vi "ziAutoRange.vi"(8 "Error in":errorcluster, 10 "Path":string, 11 "Handle in":T1 {"Handle" format="0x%08x"; "Conn" format="0x%08x"}) -> (0 "Error out":errorcluster, 1 "Success":bool, 3 "Handle out":T1 {"Handle" format="0x%08x"; "Conn" format="0x%08x"})   [LabVIEW 2009, in "Zurich Instruments LabOne.lvlib"]
doc: "Automatically set the input range of signalinputs/{0,1} to half full level.\n<B>Path</B> can either be sigins/0 or sigins/1"
uses:
  <instrlib>/Zurich Instruments LabOne/Zurich Instruments LabOne.lvlib
  <instrlib>/Zurich Instruments LabOne/Public/ziTypeHandle.ctl
  <instrlib>/Zurich Instruments LabOne/Public/Configure/ziGetValueString.vi
  <vilib>/regexp/Match Regular Expression.xnode
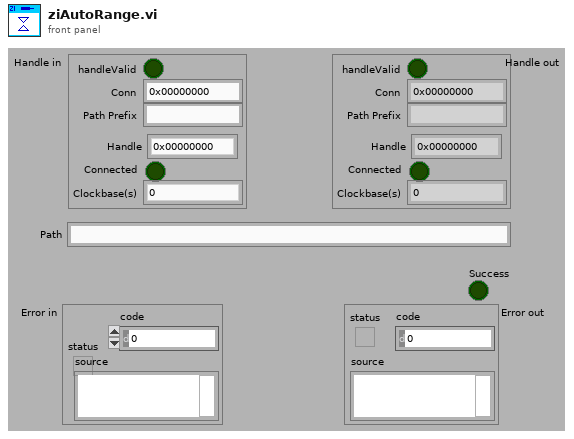
[diagram p1: front panel]
types:
  T1 = typedef "Zurich Instruments LabOne.lvlib/ziTypeHandle.ctl" = cluster{"handleValid":bool, "Conn":u64, "Path Prefix":string, "Handle":u64, "Connected":bool, "Clockbase(s)":dbl}
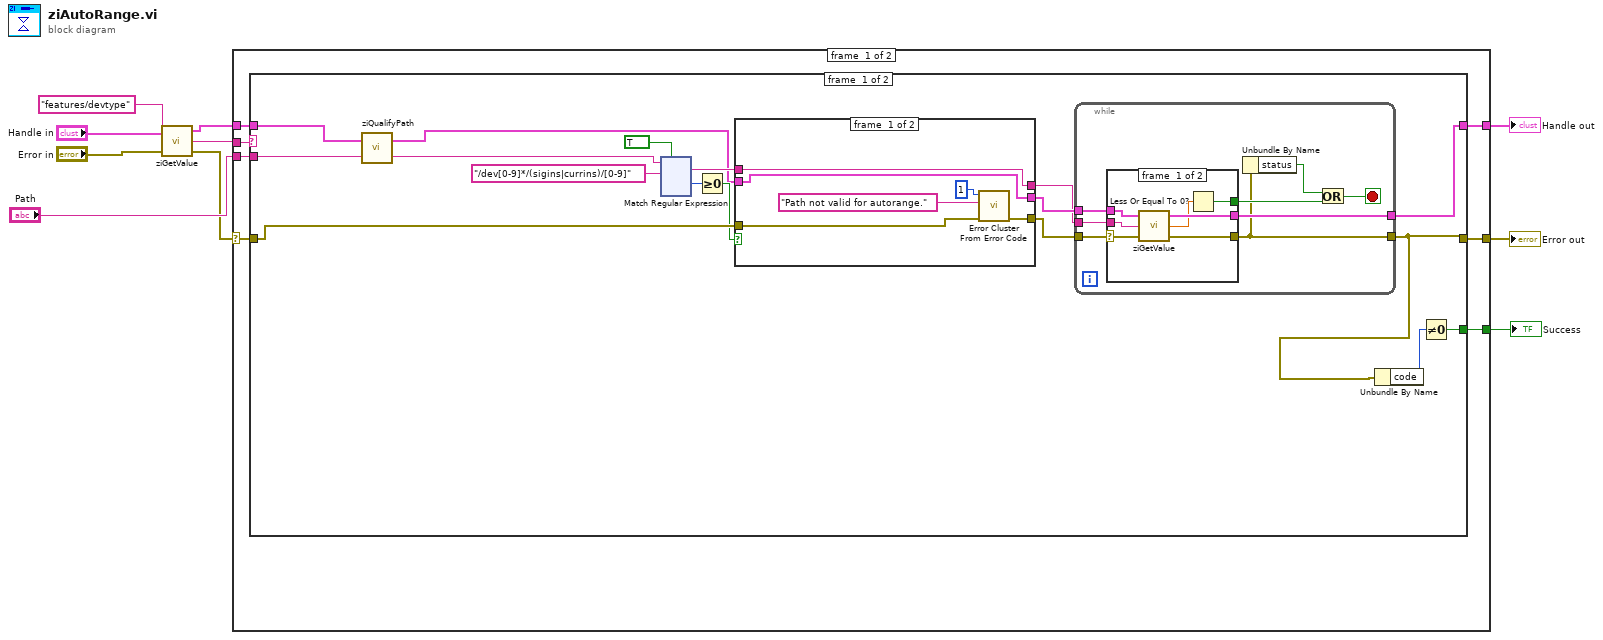
[diagram p0: block diagram]
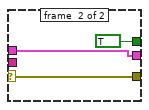
[diagram p2: hidden frame]
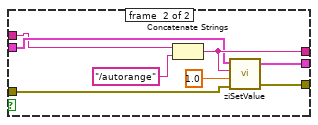
[diagram p3: hidden frame]
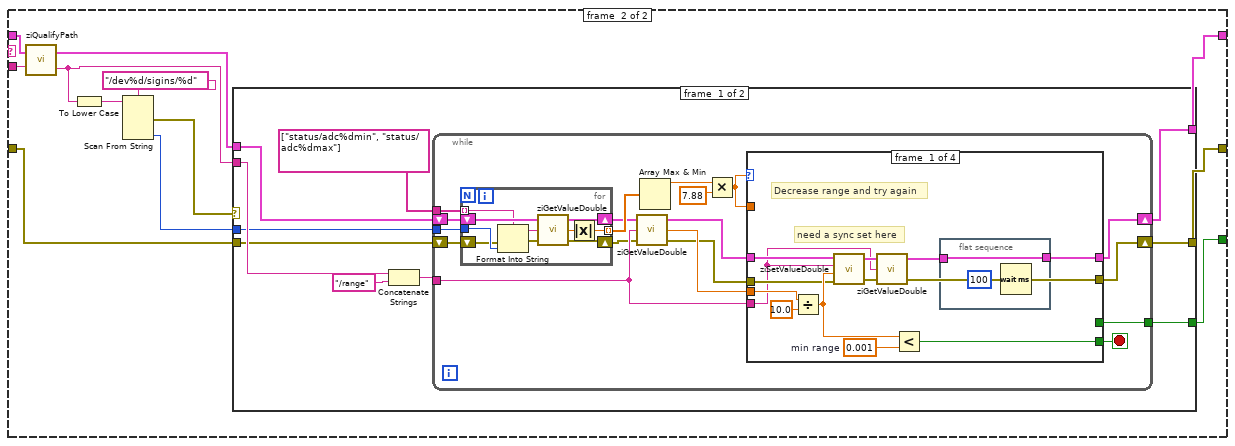
[diagram p4: hidden frame]
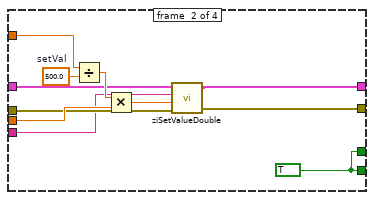
[diagram p5: hidden frame]
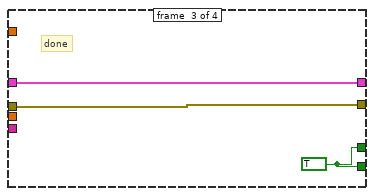
[diagram p6: hidden frame]
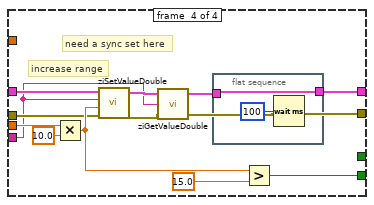
[diagram p7: hidden frame]
diagram:
  n1 = call-poly <instrlib>:"ziGetValue.vi"("error in"="Error in", "Path"="features/devtype", "Handle In"="Handle in") -> ("error out"=w2:errorcluster, "Value"=w1:string, "Handle Out"=w3:T1)
  n2 = case shown="No Error" w2 {
    selector: w2 -> [w15 w270]
    tunnel: [w17 w270] -> w10
    tunnel: [w16 w271] -> w9
    tunnel: w3 -> [w13 w271]
    tunnel: "Path" -> [w14 _]
    tunnel: [w12 _] -> w7
    tunnel: w1 -> [w11 _]
    frame #0 {
      n3 = case shown="Default" w11 {
        tunnel: [w18 w185] -> w17
        tunnel: [w32 w184] -> w16
        tunnel: w15 -> [w34 w183]
        tunnel: w14 -> [w23 w182]
        tunnel: w13 -> [w24 w181]
        tunnel: [w20 w177] -> w12
        frame #0 {
          n4 = call <instrlib>:"ziQualifyPath.vi"("Path In"=w23, "Handle In"=w24) -> ("Path Out"=w19:string, "Handle Out"=w22:T1)
          n5 = xnode "Match Regular Expression"("input string"=w19, "regular expression"="/dev[0-9]*/(sigins|currins)/[0-9]", "ignore case? (F)"=TRUE) -> ("whole match"=w29:string, "offset past match"=w27:i32)  [unwired: 3 in, 3 out]
          n6 = Greater Or Equal To 0?(x=w27) -> (x >= 0?=w28:bool)
          n7 = case shown="True" w28 {
            tunnel: w34 -> [w163 w173]
            tunnel: w22 -> [w165 w167]
            tunnel: [w165 w170] -> w33
            tunnel: [w164 w169] -> w31
            tunnel: [w162 w168] -> w30
            tunnel: w29 -> [w164 w166]
            frame #0 {
              n8 = call <vilib>:"Error Cluster From Error Code.vi"("error in (no error)"=w163, "error message (\"\")"="Path not valid for autorange." ("error message (\"\")"), "error code (0)"=1) -> ("error out"=w162:errorcluster)  [unwired: 6 in]
            }
            frame #1 {
              n9 = Concatenate Strings(w166, "/autorange") -> (w169:string)
              n10 = call-poly <instrlib>:"ziSetValue.vi"("Error In"=w173, "Value"=1.0, "Path"=w169, "Handle In"=w167) -> ("Error Out"=w168:errorcluster, "Handle Out"=w170:T1)  [unwired: 1 in]
            }
          }
          n11 = while {
            tunnel: w30 -> [w39]
            tunnel: w33 -> [w42]
            tunnel: [w41] -> w32
            tunnel: w31 -> [w40]
            tunnel: [w37] -> w18
            stop <- w35 stop-if-true
            n12 = case shown="No Error" w39 {
              selector: w39 -> [w43 w51]
              tunnel: w42 -> [w49 w52]
              tunnel: [w48 w52] -> w41
              tunnel: w40 -> [w47 _]
              tunnel: [w46 TRUE] -> w38
              tunnel: [w44 w51] -> w37
              frame #0 {
                n13 = call-poly <instrlib>:"ziGetValue.vi"("error in"=w43, "Path"=w47, "Handle in"=w49) -> ("error out"=w44:errorcluster, "Value"=w45:dbl, "Handle out"=w48:T1)
                n14 = Less Or Equal To 0?(x=w45) -> (x <= 0?=w46:bool)
              }
              frame #1 {
              }
            }
            n15 = Unbundle By Name(w37) -> ("status"=w36:bool)
            n16 = Or(x=w36, y=w38) -> (x .or. y?=w35:bool)
          }
          n17 = Unbundle By Name(w18) -> ("code"=w21:i32)
          n18 = Not Equal To 0?(x=w21) -> (x != 0?=w20:bool)
        }
        frame #1 {
          n19 = call <instrlib>:"ziQualifyPath.vi"("Path In"=w182, "Handle In"=w181) -> ("Path Out"=w176:string, "Handle Out"=w180:T1)
          n20 = To Lower Case(string=w176) -> (all lower case string=w175:string)
          n21 = Scan From String(format string="/dev%d/sigins/%d" ("regular expression"), input string=w175) -> (error out=w179:errorcluster, output 2=w174:i32)  [unwired: 5 in, 2 out]
          n22 = case shown="No Error" w179 {
            tunnel: [w192 w269] -> w185
            tunnel: [w193 w268] -> w184
            tunnel: w180 -> [w194 w268]
            tunnel: w183 -> [w186 w269]
            tunnel: w176 -> [w189 _]
            tunnel: w174 -> [w187 _]
            tunnel: [w188 _] -> w177
            frame #0 {
              n23 = Concatenate Strings(w189, "/range") -> (w191:string)
              n24 = while {
                shift-right: [w210] -> w193
                shift-left: w194 -> [w206]
                shift-right: [w209] -> w192
                shift-left: w186 -> [w198]
                tunnel: w191 -> [w201]
                tunnel: string[] ["status/adc%dmin", "status/adc%dmax"] -> [w205]
                tunnel: w187 -> [w197]
                tunnel: [w196] -> w188
                stop <- w208 stop-if-true
                n25 = for {
                  tunnel: w205 -> [w218] mode=indexing
                  tunnel: [w223] -> w213 mode=indexing
                  shift-right: [w222] -> w204
                  shift-left: w206 -> [w221]
                  tunnel: w197 -> [w217]
                  shift-right: [w219] -> w199
                  shift-left: w198 -> [w215]
                  n26 = Format Into String(format string=w218, error in=w215, w217) -> (resulting string=w216:string, error out=w214:errorcluster)  [unwired: 1 in]
                  n27 = call <instrlib>:"ziGetValueDouble.vi"("error in"=w214, "Path"=w216, "Handle in"=w221) -> ("error out"=w219:errorcluster, "Value"=w220:dbl, "Handle out"=w222:T1)
                  n28 = Absolute Value(x=w220) -> (abs(x)=w223:dbl)
                }
                n29 = call <instrlib>:"ziGetValueDouble.vi"("error in"=w199, "Path"=w201, "Handle in"=w204) -> ("error out"=w200:errorcluster, "Value"=w202:dbl, "Handle out"=w203:T1)
                n30 = Array Max & Min(array=w213) -> (max value=w211:dbl)  [unwired: 3 out]
                n31 = Multiply(x=w211, y=7.88 ("valueD")) -> (x*y=w207:dbl)
                n32 = case shown="1000..10000" w207 {
                  tunnel: w203 -> [w233 w243 w251 w261]
                  tunnel: w200 -> [w231 w241 w252 w259]
                  tunnel: [w226 w245 w251 w255] -> w210
                  tunnel: [w225 w244 w252 w254] -> w209
                  tunnel: [w224 w239 w250 w262] -> w208
                  tunnel: w202 -> [w236 w249 _ w264]
                  tunnel: w207 -> [_ w247 _ _]
                  tunnel: w201 -> [w229 w240 _ w253]
                  tunnel: [_ w239 w250 _] -> w196
                  frame #0 {
                    w234 = 0.001  # min range
                    # "need a sync set here"
                    # "Decrease range and try again"
                    n33 = Divide(x=w236, y=10.0 ("valueD")) -> (x/y=w232:dbl)
                    n34 = call <instrlib>:"ziSetValueDouble.vi"("Error In"=w231, "Value"=w232, "Path"=w229, "Handle In"=w233) -> ("Error Out"=w228:errorcluster, "Handle Out"=w230:T1)  [unwired: 1 in]
                    n35 = call <instrlib>:"ziGetValueDouble.vi"("error in"=w228, "Path"=w229, "Handle in"=w230) -> ("error out"=w225:errorcluster, "Handle out"=w227:T1)  [unwired: 1 out]
                    n36 = Less?(x=w232, y=w234) -> (x < y?=w224:bool)
                    n37 = flat-sequence {
                      tunnel: w227 -> [w237]
                      tunnel: [w237] -> w226
                      frame #0 {
                        n38 = Wait (ms)(milliseconds to wait=u32 100) -> ()  [unwired: 1 out]
                      }
                    }
                  }
                  frame #1 {
                    w246 = 500.0  # setVal
                    w239 = TRUE
                    n39 = Divide(x=w247, y=w246) -> (x/y=w248:dbl)
                    n40 = Multiply(x=w248, y=w249) -> (x*y=w242:dbl)
                    n41 = call <instrlib>:"ziSetValueDouble.vi"("Error In"=w241, "Value"=w242, "Path"=w240, "Handle In"=w243) -> ("Error Out"=w244:errorcluster, "Handle Out"=w245:T1)  [unwired: 1 in]
                  }
                  frame #2 {
                    w250 = TRUE
                    # "done"
                  }
                  frame #3 {
                    # "need a sync set here"
                    # "increase range"
                    n42 = Multiply(x=w264, y=10.0 ("valueD")) -> (x*y=w260:dbl)
                    n43 = call <instrlib>:"ziSetValueDouble.vi"("Error In"=w259, "Value"=w260, "Path"=w253, "Handle In"=w261) -> ("Error Out"=w257:errorcluster, "Handle Out"=w258:T1)  [unwired: 1 in]
                    n44 = call <instrlib>:"ziGetValueDouble.vi"("error in"=w257, "Path"=w253, "Handle in"=w258) -> ("error out"=w254:errorcluster, "Handle out"=w256:T1)  [unwired: 1 out]
                    n45 = flat-sequence {
                      tunnel: w256 -> [w266]
                      tunnel: [w266] -> w255
                      frame #0 {
                        n46 = Wait (ms)(milliseconds to wait=u32 100) -> ()  [unwired: 1 out]
                      }
                    }
                    n47 = Greater?(x=w260, y=15.0 ("valueD")) -> (0:w262:bool)
                  }
                }
              }
            }
            frame #1 {
            }
          }
        }
      }
    }
    frame #1 {
    }
  }
  "Handle out" <- w9
  "Error out" <- w10
  "Success" <- w7
